vi "Odonew.vi"(4 "Arrastrado":dbl[](array[numeric]), 5 "l":dbl, 6 "Paso":dbl, 7 "r":dbl, 9 "PA":dbl[](array[numeric]), 10 "phiL":dbl, 11 "phiR":dbl) -> (2 "Velocidad actual":dbl[](array[numeric]), 3 "Posición actual":dbl[](array[numeric]))   [LabVIEW 2011]
uses:
  <vilib>/Analysis/Matrix/Datatypes/RealMatrix.ctl
  <vilib>/Analysis/_algsub.llb/Real PseudoInverse Matrix.vi
  <vilib>/Analysis/baseanly.llb/Real A x B.vi
  <vilib>/Analysis/Matrix/NI_Matrix.lvlib
  <vilib>/Analysis/NI_AALBase.lvlib
  <vilib>/Analysis/NI_AALPro.lvlib
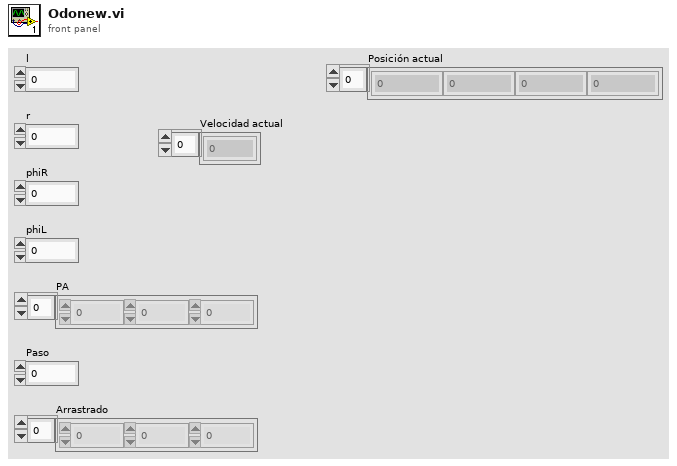
[diagram p1: front panel]
types:
  T1 = typedef "NI_Matrix.lvlib/RealMatrix.ctl" = dbl[][]
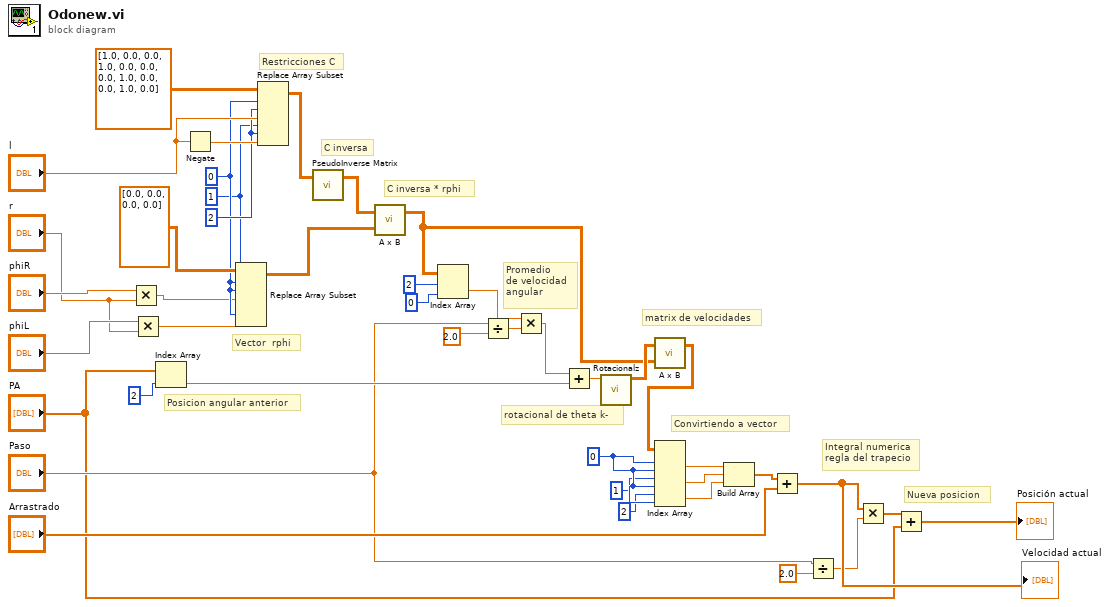
[diagram p0: block diagram]
diagram:
  w15 = 0 ("index (row)")
  w32 = 1
  w33 = 0
  w38 = 2
  # "Promedio \nde velocidad \nangular"
  # "Posicion angular anterior"
  # "Nueva posicion"
  # "Integral numerica\nregla del trapecio"
  # "Convirtiendo a vector"
  # "matrix de velocidades"
  # "rotacional de theta k-"
  # "Vector  rphi"
  # "C inversa * rphi"
  # "Restricciones C"
  # "C inversa"
  n1 = Multiply(x="phiR", y="r") -> (x*y=w24:dbl)
  n2 = Multiply(x="phiL", y="r") -> (x*y=w25:dbl)
  n3 = Index Array(array="PA", index=2) -> (element=w19:dbl)
  n4 = Negate(x="l") -> (-x=w40:dbl)
  n5 = Replace Array Subset(array=T1 [[0.0], [0.0], [0.0], [0.0]] ("Real Matrix"), new element #1=w24, index (row) #1=w33, index (col) #1=w33, new element #2=w25, index (row) #2=w32, index (col) #2=w33) -> (w30:T1)
  n6 = Replace Array Subset(array=T1 [[1.0, 0.0, 0.0], [1.0, 0.0, 0.0], [0.0, 1.0, 0.0], [0.0, 1.0, 0.0]] ("Real Matrix"), new element #1="l", index (row) #1=w33, index (col) #1=w38, new element #2=w40, index (row) #2=w32, index (col) #2=w38) -> (w31:T1)
  n7 = call-poly <vilib>:"PseudoInverse Matrix.vi"("Input Matrix"=w31) -> ("PseudoInverse Matrix"=w29:T1)  [unwired: 1 in, 1 out]
  n8 = call-poly <vilib>:"A x B.vi"("B"=w30, "A"=w29) -> ("A x B"=w16:T1)  [unwired: 1 out]
  n9 = Index Array(array=w16, index (row)=2 ("index (col)"), index (col)=0) -> (element=w21:dbl)
  n10 = Divide(x="Paso", y=2.0) -> (x/y=w22:dbl)
  n11 = Multiply(x=w21, y=w22) -> (x*y=w20:dbl)
  n12 = Add(x=w20, y=w19) -> (x+y=w18:dbl)
  n13 = call "Rotacionalz.vi"("theta"=w18) -> ("Real Matrix"=w17:T1)  [unwired: 10 in]
  n14 = call-poly <vilib>:"A x B.vi"("B"=w16, "A"=w17) -> ("A x B"=w12:T1)  [unwired: 1 out]
  n15 = Index Array ("Get Matrix Elements")(array=w12, index (row) #1=w15, index (col) #1=w15, index (row) #2=1 ("index (row)"), index (col) #2=w15, index (row) #3=2 ("index (row)"), index (col) #3=w15) -> (element #1=w9:dbl, element #2=w10:dbl, element #3=w11:dbl)
  n16 = Build Array(w9, w10, w11) -> (w8:dbl[])
  n17 = Add(x=w8, y="Arrastrado") -> (x+y=w42:dbl[])
  "Velocidad actual" <- w42
  n18 = Divide(x="Paso", y=2.0) -> (x/y=w4:dbl)
  n19 = Multiply(x=w42, y=w4) -> (x*y=w3:dbl[])
  n20 = Add(x=w3, y="PA") -> (x+y=→"Posición actual":dbl[])
